vi "N DBL to Result.vi"(8 "error in (no error)":errorcluster, 9 "Data":dbl[](array[numeric]), 10 "Result in":refnum<class "Acquired Result.lvclass">, 11 "Instrument Driver in":refnum<class "Instrument Driver.lvclass">) -> (0 "error out":errorcluster, 2 "Result out":refnum<class "Acquired Result.lvclass">, 3 "Instrument Driver out":refnum<class "Instrument Driver.lvclass">)   [LabVIEW 2019, in "Instrument Driver.lvclass"]
uses:
  Instrument Driver.lvclass
  <vilib>/express/express shared/transition.llb/Dynamic To Waveform Array.vi
  <vilib>/express/express signal manip/GetorSetDDTAttributes/Set DDT Attributes/SetT0.vi
  <vilib>/express/express shared/transition.llb/Waveform Array To Dynamic.vi
  <vilib>/express/express signal manip/GetorSetDDTAttributes/Set DDT Attributes/Set DDT Properties.xnode
  Results/Acquired Result/Acquired Result.lvclass
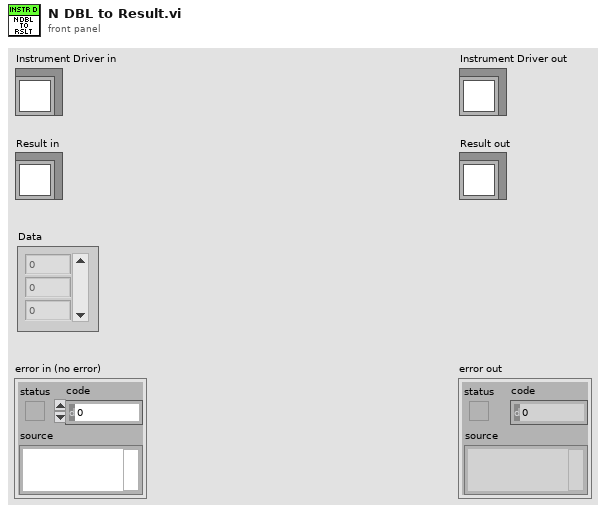
[diagram p1: front panel]
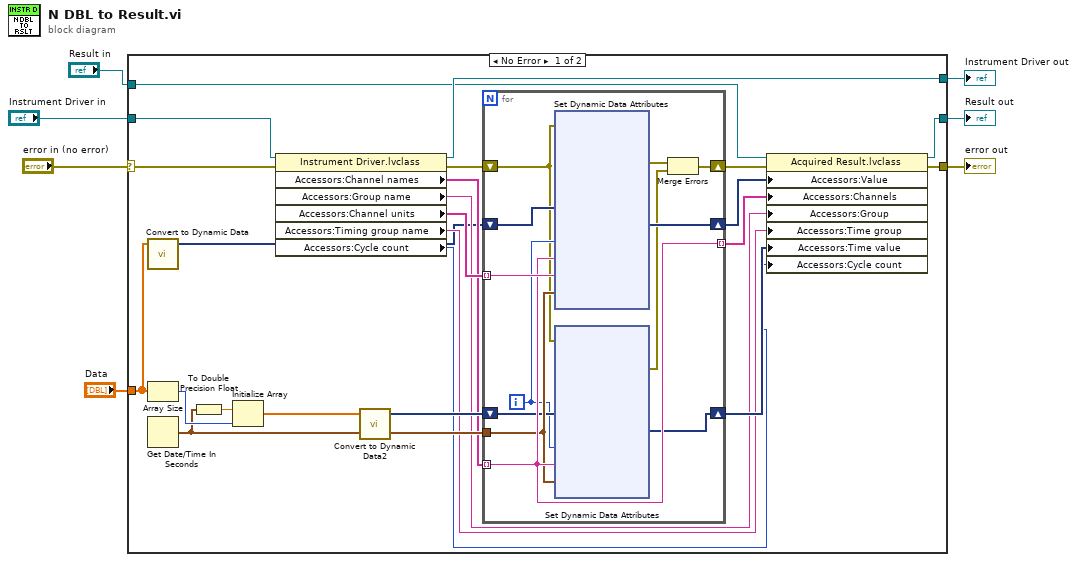
[diagram p0: block diagram]
diagram:
  n1 = case shown="No Error" "error in (no error)" {
    selector: "error in (no error)" -> [w15 w83]
    tunnel: [w12 w83] -> w6
    tunnel: [w10 w82] -> w4
    tunnel: "Instrument Driver in" -> [w11 w82]
    tunnel: "Data" -> [w14 _]
    tunnel: [w13 w81] -> w2
    tunnel: "Result in" -> [w9 w81]
    frame No Error {
      n2 = call "Convert to Dynamic Data"("Array"=w14) -> ("Dynamic Data Type"=w17:dynamicdata)  [unwired: 3 in]
      n3 = Array Size(array=w14) -> (size(s)=w30:i32)
      n4 = Get Date/Time In Seconds() -> (seconds since 1Jan1904=w25:timestamp)
      n5 = To Double Precision Float(number=w25) -> (double precision float=w26:dbl)
      n6 = Initialize Array(w26, w30) -> (w27:dbl[])
      n7 = property class="Instrument Driver.lvclass"(reference=w11, error in=w15) -> (reference out=w10:refnum<class "Instrument Driver.lvclass">, error out=w23:errorcluster, "Accessors:Channel names"=w20:string[], "Accessors:Group name"=w21:string, "Accessors:Channel units"=w22:string[], "Accessors:Timing group name"=w24:string, "Accessors:Cycle count"=w8:i32)
      n8 = call "Convert to Dynamic Data2"("Array"=w27) -> ("Dynamic Data Type"=w28:dynamicdata)  [unwired: 3 in]
      n9 = for {
        tunnel: [w38] -> w19 mode=indexing
        tunnel: w20 -> [w38] mode=indexing
        tunnel: w22 -> [w39] mode=indexing
        shift-right: [w40] -> w16
        shift-left: w17 -> [w41]
        shift-right: [w32] -> w18
        shift-left: w23 -> [w33]
        tunnel: w25 -> [w37]
        shift-right: [w34] -> w29
        shift-left: w28 -> [w36]
        i -> [w35]
        n10 = xnode "Set Dynamic Data Attributes"("Signals In"=w41, "Signal Index"=w35, "Signal Name"=w38, "Unit"=w39, "Timestamp"=w37, "error in"=w33) -> ("Signals Out"=w40:dynamicdata, "error out"=w42:errorcluster)
        n11 = xnode "Set Dynamic Data Attributes"("Signals In"=w36, "Signal Index"=w35, "Signal Name"=w38, "Timestamp"=w37, "error in"=w33) -> ("Signals Out"=w34:dynamicdata, "error out"=w31:errorcluster)
        n12 = Merge Errors(w42, w31) -> (w32:errorcluster)
      }
      n13 = property class="Acquired Result.lvclass"(reference=w9, error in=w18, "Accessors:Value"=w16, "Accessors:Channels"=w19, "Accessors:Group"=w21, "Accessors:Time group"=w24, "Accessors:Time value"=w29, "Accessors:Cycle count"=w8) -> (reference out=w13:refnum<class "Acquired Result.lvclass">, error out=w12:errorcluster)
    }
    frame Error {
    }
  }
  "error out" <- w6
  "Instrument Driver out" <- w4
  "Result out" <- w2
